vi "DemoClass1_New.vi"(0 "reference in":refnum<class "DemoClass1.lvclass">, 1 "Object name":string, 5 "error in (no error)":errorcluster, 7 "User counter":bool, 8 "Create method":T1(ring)) -> (14 "reference out":refnum<class "DemoClass1.lvclass">, 16 "# of objects":i32, 17 "First user":bool, 19 "error out":errorcluster)   [LabVIEW 2016, in "DemoClass1.lvclass"]
doc: "Looks up an existing object matching object name or creates a new object and returns a refnum you can use when calling other class methods.\n\nObjects created with this VI should be destroyed using this class Delete VI."
uses:
  <vilib>/addons/GOOPUtility/_Demo/GOOPUtil_Demo/DemoClass1_class/DemoClass1.lvclass
  <vilib>/addons/_goop3.llb/3GOOPStates.ctl
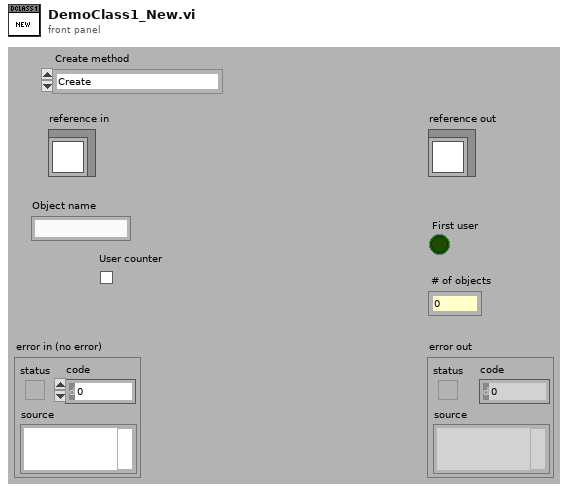
[diagram p1: front panel]
types:
  T1 = enum16{"Create", "Create or look up existing", "Look up existing"}
  T2 = typedef "3GOOPStates.ctl" = enum16{"Set", "Get", "New", "Delete", "Clear", "Test and get", "Unlock data", "Information", "Look up existing", "New or look up existing", "Test and get shared", "Get shared", "Set shared", "Unlock shared", "Find dynamic method", "Register dynamic method", "Preload dynamic method", "Probe", "Cast to more generic", "Cast to more specific"}
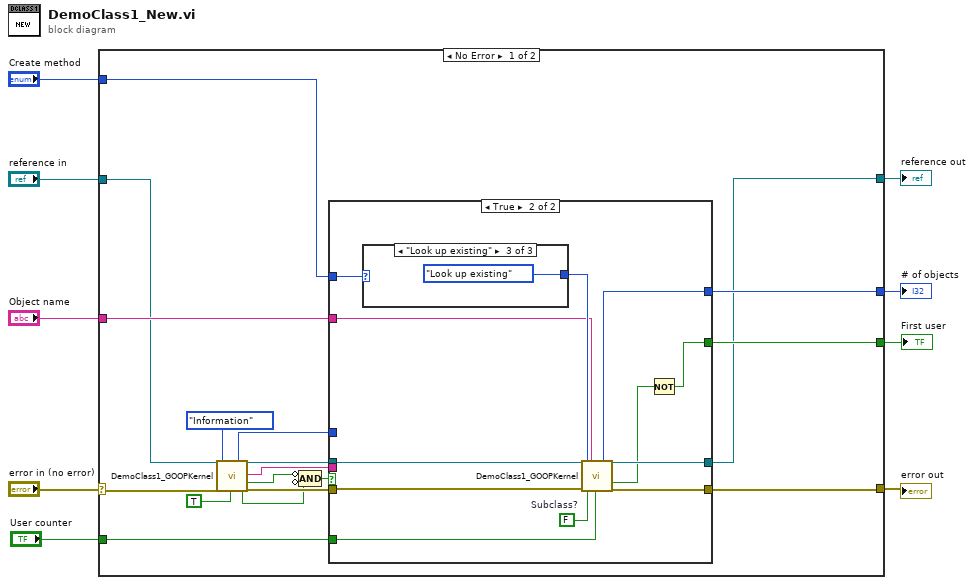
[diagram p0: block diagram]
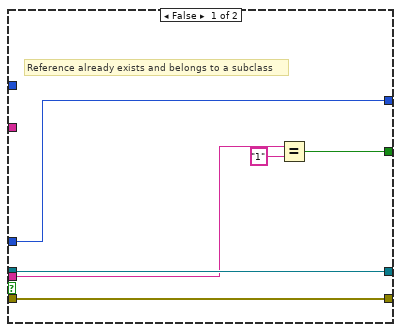
[diagram p2: hidden frame]
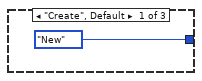
[diagram p3: hidden frame]
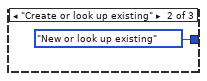
[diagram p4: hidden frame]
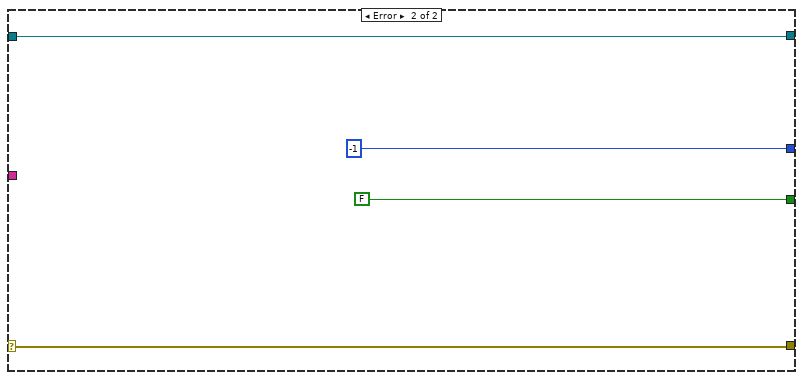
[diagram p5: hidden frame]
diagram:
  n1 = case shown="No Error" "error in (no error)" {
    selector: "error in (no error)" -> [w24 w51]
    tunnel: [w27 w51] -> w9
    tunnel: [w26 -1 ("Nr of open handles")] -> w8
    tunnel: "Object name" -> [w25 _]
    tunnel: "Create method" -> [w16 _]
    tunnel: "reference in" -> [w11 w50]
    tunnel: [w12 w50] -> w3
    tunnel: [w14 FALSE] -> w2
    tunnel: "User counter" -> [w13 _]
    frame No Error {
      n2 = call <vilib>:"DemoClass1_GOOPKernel.vi"("Ref in"=w11, "error in (no error)"=w24, "Action"=3GOOPStates."Information", "Misc"=TRUE ("First try?")) -> ("# of objects"=w19:i32, "IsSubclass?"=w22:bool, "Ref out"=w17:refnum<class "DemoClass1.lvclass">, "Probe out"=w15:string, "Exists?"=w21:bool, "error out"=w23:errorcluster)  [unwired: 13 in, 5 out]
      n3 = Compound Arithmetic op=AND(invert w21, invert w22) -> (w20:bool)
      n4 = case shown="True" w20 {
        tunnel: w16 -> [_ w45]
        tunnel: [w31 w37] -> w12
        tunnel: [w33 w44] -> w27
        tunnel: [w32 w40] -> w26
        tunnel: w25 -> [_ w41]
        tunnel: w23 -> [w33 w39]
        tunnel: w19 -> [w32 _]
        tunnel: w17 -> [w31 w38]
        tunnel: w15 -> [w29 _]
        tunnel: [w28 w35] -> w14
        tunnel: w13 -> [_ w34]
        frame False {
          # "Reference already exists and belongs to a subclass"
          n5 = Equal?(x=w29, y="1") -> (x = y?=w28:bool)
        }
        frame True {
          w42 = FALSE  # Subclass?
          n6 = case shown="\"Look up existing\"" w45 {
            tunnel: [3GOOPStates."New" ("Action") 3GOOPStates."New or look up existing" ("Action") 3GOOPStates."Look up existing" ("Action")] -> w43
            frame "Create", Default {
            }
            frame "Create or look up existing" {
            }
            frame "Look up existing" {
            }
          }
          n7 = call <vilib>:"DemoClass1_GOOPKernel.vi"("Ref in"=w38, "error in (no error)"=w39, "Action"=w43, "Subclass?"=w42, "Object name"=w41, "Misc"=w34) -> ("# of objects"=w40:i32, "Ref out"=w37:refnum<class "DemoClass1.lvclass">, "Exists?"=w36:bool, "error out"=w44:errorcluster)  [unwired: 11 in, 7 out]
          n8 = Not(x=w36) -> (.not. x?=w35:bool)
        }
      }
    }
    frame Error {
    }
  }
  "error out" <- w9
  "# of objects" <- w8
  "reference out" <- w3
  "First user" <- w2
